vi "Learn form template.vi"(8 "error in (no error)":errorcluster) -> (0 "error out":errorcluster, 3 "Refnum out":T1)   [LabVIEW 2014]
uses:
  <vilib>/vision/Image Controls.llb/IMAQ Image.ctl
  <vilib>/vision/NI_Vision_Development_Module.lvlib
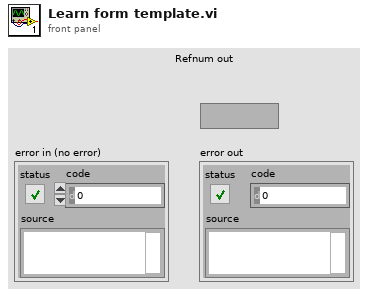
[diagram p1: front panel]
types:
  T1 = typedef "IMAQ Image.ctl" = refnum<image>
  T2 = typedef "Image Type" = u32
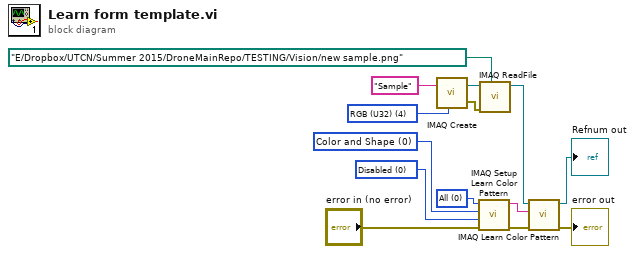
[diagram p0: block diagram]
diagram:
  w9 = T2 4 items=["Grayscale (U8)", "Grayscale (I16)", "Grayscale (SGL)", "Complex (CSG)", "RGB (U32)", "HSL (U32)", "RGB (U64)", "Grayscale (U16)"] ("Image Type")
  w4 = u32 0 items=["Disabled", "Ignore Black", "Ignore White", "Ignore Black and White"] ("Ignore Black and White")
  w3 = u32 0 items=["Color and Shape", "Color", "Shape "] ("Feature Mode")
  w2 = u32 0 items=["All", "Shift Information", "Rotation Information"] ("Learn Mode")
  n1 = call "IMAQ Create"("Image Name"="Sample", "Image Type"=w9) -> ("New Image"=w10:T1, "error out"=w7:errorcluster)  [unwired: 3 in]
  n2 = call "IMAQ Setup Learn Color Pattern"("error in (no error)"="error in (no error)", "Ignore Black and White"=w4, "Feature Mode"=w3, "Learn Mode"=w2) -> ("error out"=w1:errorcluster, "Learn Color Pattern Setup Data"=w5:string)  [unwired: 6 in]
  n3 = call "IMAQ ReadFile"("File Path"=path "E:/Dropbox/UTCN/Summer 2015/DroneMainRepo/TESTING/Vision/new sample.png", "error in (no error)"=w7, "Image"=w10) -> ("Image Out"=w11:T1)  [unwired: 4 in, 4 out]
  n4 = call "IMAQ Learn Color Pattern"("error in (no error)"=w1, "Learn Color Pattern Setup Data"=w5, "Image"=w11) -> ("error out"=→"error out":errorcluster, "Template Image Out"=→"Refnum out":T1)  [unwired: 7 in]
